vi "Configure Control AI Filter.vi"(0 "VISA resource name":refnum<visa-resource-name>, 1 "Delay Time":i32=1 min=0 max=120, 5 "Unit No. (0)":i32 min=0 max=6, 7 "Module No.(0)":i32 min=0 max=9, 9 "AI No.(1)":i32=1 min=1 max=2, 11 "error in (no error)":errorcluster, 12 "Used flag(false)":bool) -> (4 "VISA resource name out":refnum<visa-resource-name>, 6 "AI No.":i32, 8 "Unit No.":i32, 10 "Module No.":i32, 15 "error out":errorcluster)   [LabVIEW 2020, in "Yokogawa GX Series.lvlib"]
doc: "Set the first-order lag filter of the AI channel of the PID module\n\nCommand: SCtrlFilter"
uses:
  <instrlib>/Yokogawa GX Series/Yokogawa GX Series.lvlib
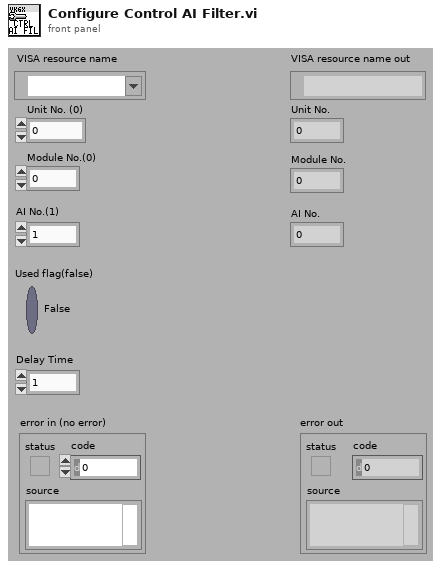
[diagram p1: front panel]
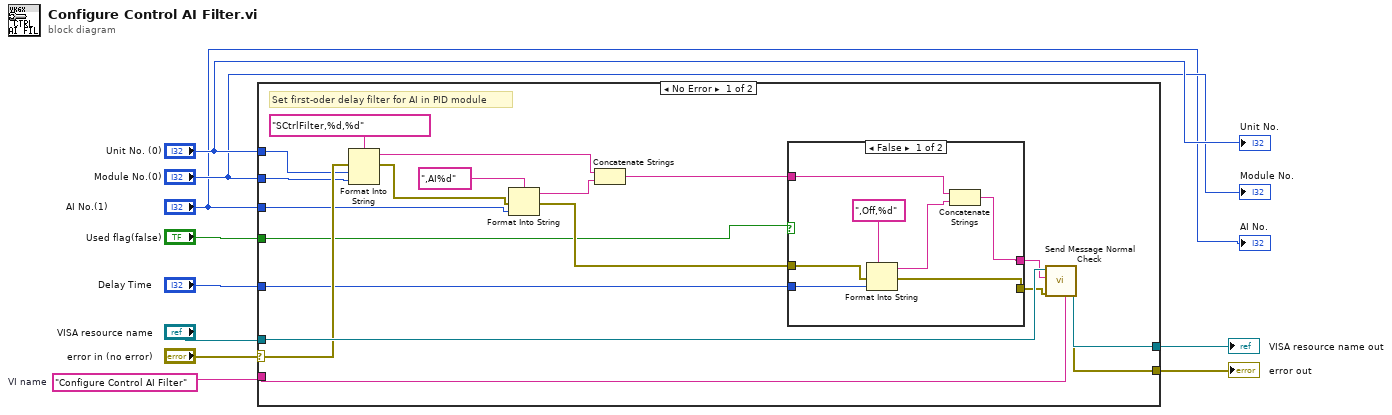
[diagram p0: block diagram]
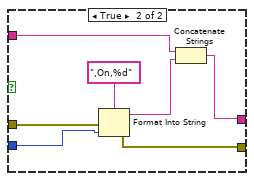
[diagram p2: hidden frame]
diagram:
  w6 = "Configure Control AI Filter"  # VI name
  n1 = case shown="No Error" "error in (no error)" {
    selector: "error in (no error)" -> [w25 w44]
    tunnel: [w29 w45] -> w10
    tunnel: [w28 w44] -> w9
    tunnel: "VISA resource name" -> [w27 w45]
    tunnel: w6 -> [w24 _]
    tunnel: "Unit No. (0)" -> [w23 _]
    tunnel: "Module No.(0)" -> [w22 _]
    tunnel: "AI No.(1)" -> [w20 _]
    tunnel: "Delay Time" -> [w13 _]
    tunnel: "Used flag(false)" -> [w12 _]
    frame No Error {
      # "Set first-oder delay filter for AI in PID module"
      n2 = Format Into String(format string="SCtrlFilter,%d,%d", error in=w25, w23, w22) -> (resulting string=w18:string, error out=w19:errorcluster)  [unwired: 1 in]
      n3 = Format Into String(format string=",AI%d", error in=w19, w20) -> (resulting string=w17:string, error out=w15:errorcluster)  [unwired: 1 in]
      n4 = Concatenate Strings(w18, w17) -> (w11:string)
      n5 = case shown="False" w12 {
        tunnel: [w35 w38] -> w16
        tunnel: w15 -> [w31 w42]
        tunnel: [w30 w41] -> w14
        tunnel: w13 -> [w33 w40]
        tunnel: w11 -> [w36 w37]
        frame False {
          n6 = Format Into String(format string=",Off,%d", error in=w31, w33) -> (resulting string=w32:string, error out=w30:errorcluster)  [unwired: 1 in]
          n7 = Concatenate Strings(w36, w32) -> (w35:string)
        }
        frame True {
          n8 = Format Into String(format string=",On,%d", error in=w42, w40) -> (resulting string=w39:string, error out=w41:errorcluster)  [unwired: 1 in]
          n9 = Concatenate Strings(w37, w39) -> (w38:string)
        }
      }
      n10 = call <instrlib>:"Send Message Normal Check.vi"("Source (\"\")"=w24, "error in (no error)"=w14, "Send Message (\"\")"=w16, "VISA resource name"=w27) -> ("error out"=w28:errorcluster, "VISA resource name out"=w29:refnum<visa-resource-name>)  [unwired: 2 in, 4 out]
    }
    frame Error {
    }
  }
  "error out" <- w9
  "VISA resource name out" <- w10
  "Unit No." <- "Unit No. (0)"
  "Module No." <- "Module No.(0)"
  "AI No." <- "AI No.(1)"
